vi "lab session 6.2.vi"() -> ()   [LabVIEW 2020]
panel:
  out "iteration":i32
  out "Array":dbl[](array[numeric])
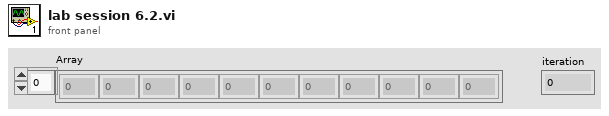
[diagram p1: front panel]
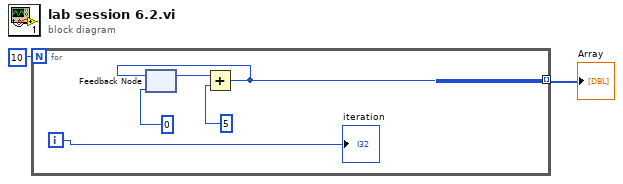
[diagram p0: block diagram]
diagram:
  n1 = for {
    N: 10 -> [_]
    tunnel: [w5] -> w1 mode=indexing
    i -> [w3]
    n2 = feedback #1(0) -> (w6:i32)
    n3 = Add(x=w6, y=5) -> (x+y=w5:i32)
    n4 = feedback-in #1(w5) -> ()
    "iteration" <- w3
  }
  "Array" <- w1
